vi "Benchmark SV Receive LV2012 - NI Verified - 10 Byte - PC - 1Var.vi"() -> ()   [LabVIEW 2015]
panel:
  out "Average Delay (ms)":dbl
  out "Delay (ms)":u32
  out "Counter":i32
  in  "10 byte 2":u64[][](array[numeric])=[[0, 0, 0, 0, 0, 0, 0, 0, 0, 0], [0, 0, 0, 0, 0, 0, 0, 0, 0, 0]]
  out "appended array":u64[][](array[numeric])
  out "10 byte":u64[](array[numeric])
  in  "stop":bool
  # "Overview:  Coding that exemplifies how to benchmark the communication of Shared Variables.\nRequirements: LabVIEW 2012 or compatible\nInstructions:\n1. Run this VI\n2. Watch the amount of time it takes to communicate on the \"Benchmark SV Send  LV2012 - NI Verified.vi\" \n3. Stop both VIs"
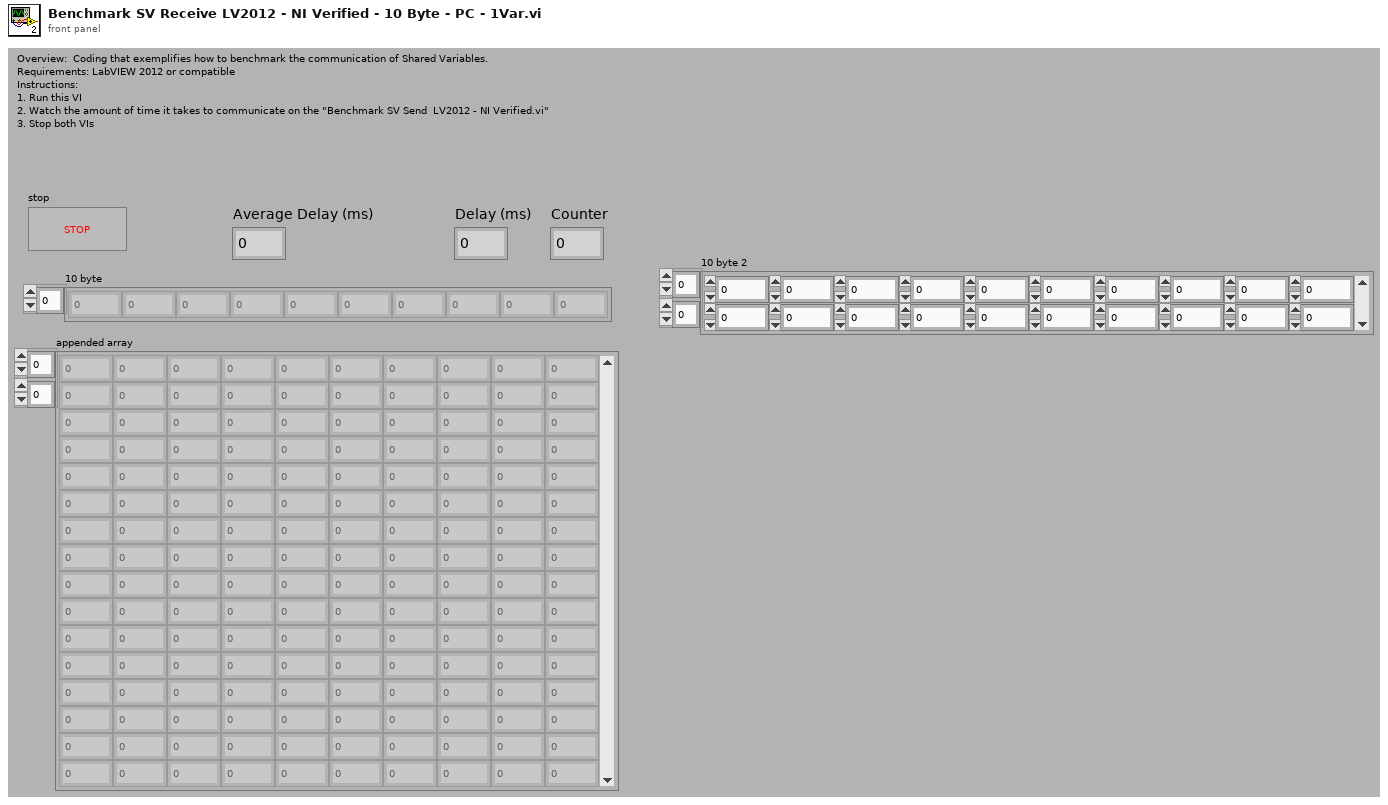
[diagram p1: front panel]
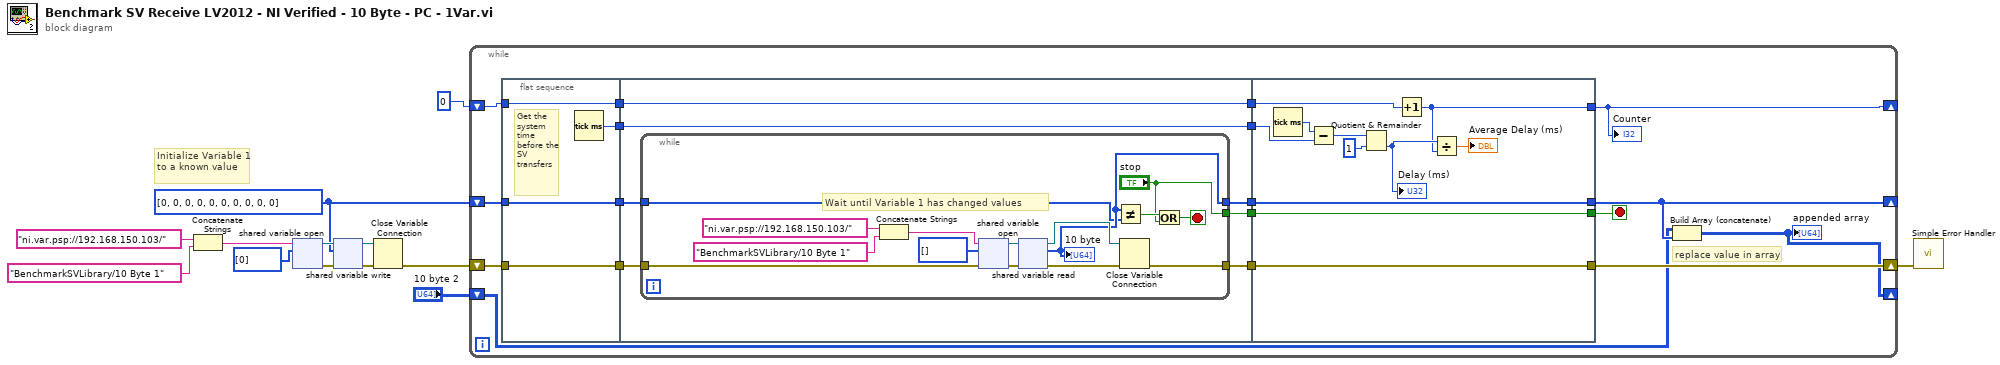
[diagram p0: block diagram]
diagram:
  w3 = u64[] [0, 0, 0, 0, 0, 0, 0, 0, 0, 0] ("appended array")
  # "Initialize Variable 1 to a known value"
  n1 = Concatenate Strings("ni.var.psp://192.168.150.103/" ("string"), "BenchmarkSVLibrary/10 Byte 1") -> (w12:string)
  n2 = shared-variable-open(w12, u64[] [0] ("appended array")) -> (w10:refnum<k21>, w8:errorcluster)  [unwired: 2 in]
  n3 = shared-variable-write(w10, w8, w3) -> (w9:refnum<k21>, w7:errorcluster)
  n4 = Close Variable Connection(8:w7, 11:w9) -> (0:w6:errorcluster)
  n5 = while {
    shift-right: [w27] -> _
    shift-left: w3 -> [w31]
    shift-right: [w29] -> w13
    shift-left: w6 -> [w30]
    shift-right: [w26] -> _
    shift-left: "10 byte 2" -> [w25]
    shift-right: [w14] -> _
    shift-left: 0 -> [w16]
    stop <- w28 stop-if-true
    # "replace value in array"
    n6 = flat-sequence {
      tunnel: w30 -> [w34]
      tunnel: w31 -> [w35]
      tunnel: [w35] -> w24
      tunnel: [w34] -> w23
      tunnel: [w33] -> w18
      tunnel: [w32] -> w17
      tunnel: w16 -> [w32]
      tunnel: w24 -> [w42]
      tunnel: w23 -> [w41]
      tunnel: [w40] -> w22
      tunnel: [w39] -> w21
      tunnel: [w38] -> w20
      tunnel: [w37] -> w19
      tunnel: w18 -> [w37]
      tunnel: w17 -> [w36]
      tunnel: [w36] -> w15
      tunnel: [w66] -> w27
      tunnel: [w67] -> w28
      tunnel: [w68] -> w29
      tunnel: w22 -> [w68]
      tunnel: w21 -> [w67]
      tunnel: w20 -> [w66]
      tunnel: w19 -> [w61]
      tunnel: w15 -> [w59]
      tunnel: [w58] -> w14
      frame #0 {
        # "Get the system time before the SV transfers"
        n7 = Tick Count (ms)() -> (millisecond timer value=w33:u32)
      }
      frame #1 {
        n8 = while {
          tunnel: w42 -> [w43]
          tunnel: [w44] -> w38
          tunnel: ["stop"] -> w39
          tunnel: [w49] -> w40
          tunnel: w41 -> [w48]
          stop <- w55 stop-if-true
          # "Wait until Variable 1 has changed values"
          n9 = Concatenate Strings("ni.var.psp://192.168.150.103/" ("string"), "BenchmarkSVLibrary/10 Byte 1") -> (w45:string)
          n10 = shared-variable-open(w45, w48, u64[] [] ("appended array")) -> (w53:refnum<k21>, w52:errorcluster)  [unwired: 1 in]
          n11 = shared-variable-read(w53, w52) -> (w51:refnum<k21>, w50:errorcluster, w44:u64[])  [unwired: 1 out]
          "10 byte" <- w44
          n12 = Not Equal?(x=w44, y=w43) -> (x != y?=w57:bool)
          n13 = Close Variable Connection(8:w50, 11:w51) -> (0:w49:errorcluster)
          n14 = Or(x=w57, y="stop") -> (x .or. y?=w55:bool)
        }
      }
      frame #2 {
        n15 = Tick Count (ms)() -> (millisecond timer value=w62:u32)
        n16 = Subtract(x=w62, y=w61) -> (x-y=w63:u32)
        n17 = Quotient & Remainder(x=w63, y=u32 1) -> (floor(x/y)=w65:u32)  [unwired: 1 out]
        "Delay (ms)" <- w65
        n18 = Increment(x=w59) -> (x+1=w58:i32)
        n19 = Divide(x=w65, y=w58) -> (x/y=→"Average Delay (ms)":dbl)
      }
    }
    n20 = Build Array (concatenate)(w25, w27) -> (w26:u64[][])
    "appended array" <- w26
    "Counter" <- w14
  }
  n21 = call <vilib>:"Simple Error Handler.vi"("error in (no error)"=w13) -> ()  [unwired: 4 in, 5 out]
